vi "Determine Archive Types.vi"(2 "2 LBCB Archiving Mode":bool, 3 "Number of\nLBCBs Out":T2) -> (0 "Response Archive Types":T1[](array[typedef]), 1 "Command & Stiffness Types":T1[](array[typedef]))   [LabVIEW 2009]
uses:
  Archive File Type.ctl
  Data Access Objects/Application/Number Of LBCBs.ctl
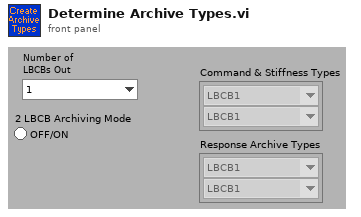
[diagram p1: front panel]
types:
  T1 = typedef "Archive File Type.ctl" = enum16{"LBCB1", "LBCB2", "ExternalSensors", "Combined"}
  T2 = typedef "Number Of LBCBs.ctl" = enum16{"1", "2"}
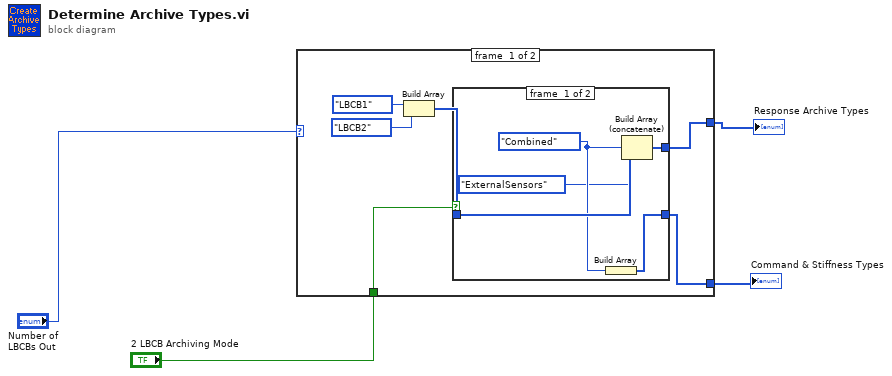
[diagram p0: block diagram]
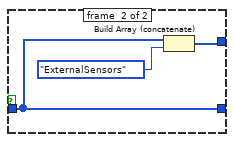
[diagram p2: hidden frame]
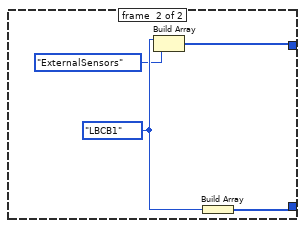
[diagram p3: hidden frame]
diagram:
  n1 = case shown="\"2\"" "Number of\nLBCBs Out" {
    tunnel: "2 LBCB Archiving Mode" -> [w10 _]
    tunnel: [w6 w20] -> w2
    tunnel: [w5 w19] -> w4
    frame #0 {
      n2 = Build Array(Archive_File_Type."LBCB1" ("Archive File Type"), Archive_File_Type."LBCB2" ("element")) -> (w8:T1[])
      n3 = case shown="True" w10 {
        tunnel: w8 -> [w15 w18]
        tunnel: [w12 w16] -> w6
        tunnel: [w11 w18] -> w5
        frame #0 {
          w14 = Archive_File_Type."Combined" ("element")
          n4 = Build Array(w14) -> (w11:T1[])
          n5 = Build Array (concatenate)(w15, w14, Archive_File_Type."ExternalSensors" ("element")) -> (w12:T1[])
        }
        frame #1 {
          n6 = Build Array (concatenate)(w18, Archive_File_Type."ExternalSensors" ("element")) -> (w16:T1[])
        }
      }
    }
    frame #1 {
      w22 = Archive_File_Type."LBCB1" ("Archive File Type")
      n7 = Build Array(w22, Archive_File_Type."ExternalSensors" ("element")) -> (w20:T1[])
      n8 = Build Array(w22) -> (w19:T1[])
    }
  }
  "Command & Stiffness Types" <- w4
  "Response Archive Types" <- w2
